vi "Enum indexer.vi"(9 "Step name enum in":T1=enum."Init NI", 11 "Step name":string) -> (1 "Step name enum out":T1=enum."Init NI")   [LabVIEW 2014]
uses:
  Control/Step name enum.ctl
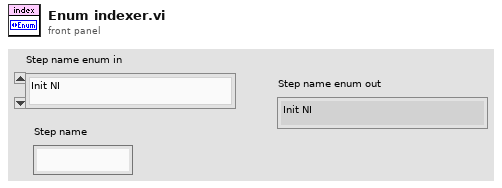
[diagram p1: front panel]
types:
  T1 = typedef "Step name enum.ctl" = enum16{"Default", "Idle", "Init Ard", "Init SM", "Init NI", "Run", "Close"}
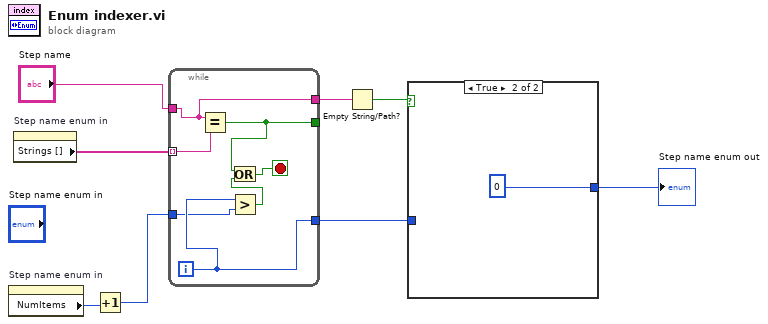
[diagram p0: block diagram]
diagram:
  n1 = property on="Step name enum in" class="Enum (strict)"() -> ("NumItems"=w2:u32)  [unwired: 2 in, 2 out]
  n2 = property on="Step name enum in" class="Enum (strict)"() -> ("Strings []"=w7:string[])  [unwired: 2 in, 2 out]
  n3 = Increment(x=w2) -> (x+1=w1:u32)
  n4 = while {
    tunnel: w7 -> [w15] mode=indexing
    tunnel: "Step name" -> [w14]
    tunnel: [w11] -> _
    tunnel: [w13] -> w3
    tunnel: [w14] -> w6
    tunnel: w1 -> [w9]
    i -> [w13]
    stop <- w10 stop-if-true
    n5 = Equal?(x=w14, y=w15) -> (x = y?=w11:bool)
    n6 = Greater?(x=w13, y=w9) -> (0:w12:bool)
    n7 = Or(x=w11, y=w12) -> (x .or. y?=w10:bool)
  }
  n8 = Empty String/Path?(string/path=w6) -> (empty?=w5:bool)
  n9 = case shown="True" w5 {
    tunnel: [w16 0] -> w4
    tunnel: w3 -> [w16 _]
    frame False {
    }
    frame True {
    }
  }
  "Step name enum out" <- w4
